vi "Set Active Worksheet.vi"(8 "error in (no error)":errorcluster, 10 "Index":i32, 11 "Report In":refnum<class "Report.lvclass">) -> (0 "error out":errorcluster, 3 "Report Out":refnum<class "Report.lvclass">)   [LabVIEW 2015, in "Report.lvclass"]
uses:
  Report.lvclass
  Report.lvclass/Report.ctl
  <vilib>/Utility/NIReport.llb/Excel/NI_Excel.lvclass
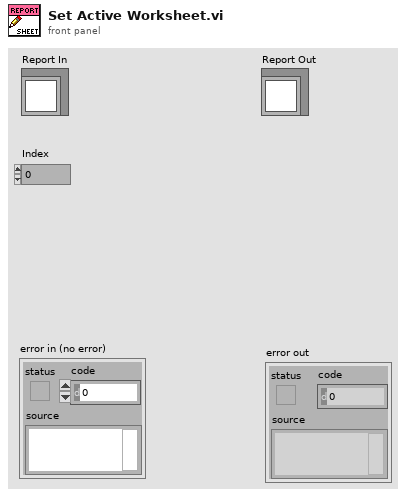
[diagram p1: front panel]
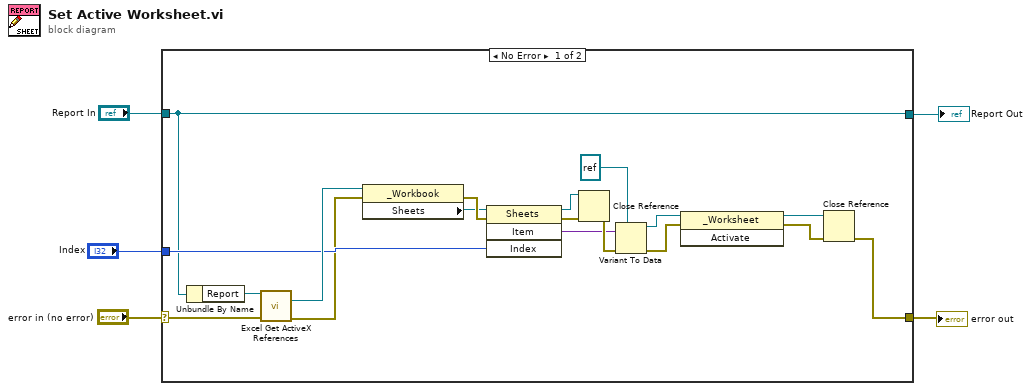
[diagram p0: block diagram]
diagram:
  n1 = case shown="No Error" "error in (no error)" {
    selector: "error in (no error)" -> [w23 w25]
    tunnel: [w7 w25] -> w5
    tunnel: "Report In" -> [w6 w24]
    tunnel: [w6 w24] -> w2
    tunnel: "Index" -> [w10 _]
    frame No Error {
      n2 = Unbundle By Name(w6) -> ("Report"=w22:refnum<class "NI_report.lvclass">)
      n3 = call <vilib>:"Excel Get ActiveX References.vi"("report in"=w22, "error in (no error)"=w23) -> ("Excel._Workbook"=w11:refnum<k7>, "error out"=w8:errorcluster)  [unwired: 7 in, 5 out]
      n4 = property class="_Workbook"(reference=w11, error in=w8) -> (error out=w19:errorcluster, "Sheets"=w18:refnum<k7>)  [unwired: 1 out]
      n5 = invoke class="Sheets" method="Item"(reference=w18, error in=w19, "Index"=w10) -> (reference out=w15:refnum<k7>, error out=w16:errorcluster, "Item"=w12:variant)  [unwired: 1 in, 1 out]
      n6 = Close Reference(reference=w15, error in (no error)=w16) -> (error out=w17:errorcluster)
      n7 = Variant To Data(error in=w17, type=refnum<k7> refnum ("Excel._Worksheet"), Variant=w12) -> (data=w14:refnum<k7>, error out=w13:errorcluster)
      n8 = invoke class="_Worksheet" method="Activate"(reference=w14, error in=w13) -> (reference out=w20:refnum<k7>, error out=w21:errorcluster)  [unwired: 1 in, 1 out]
      n9 = Close Reference(reference=w20, error in (no error)=w21) -> (error out=w7:errorcluster)
    }
    frame Error {
    }
  }
  "error out" <- w5
  "Report Out" <- w2
